vi "Sine_Trajectory.vi"(7 "Amplitude":dbl, 8 "Offset":dbl, 9 "Frequency (Hz)":dbl, 10 "Duration (s)":dbl, 11 "Period (s)":dbl) -> (3 "Profile":cluster{"time (s)":dbl, "setpoint":dbl}[](array[cluster]) {"setpoint" format="%.2f"; "time (s)" format="%.3f"})   [LabVIEW 2015]
uses:
  <vilib>/Analysis/NI_AALBase.lvlib
panel:
  out "XY Graph":cluster{dbl, dbl}[](graph)
  # "Here needs to be 0.001 or so"
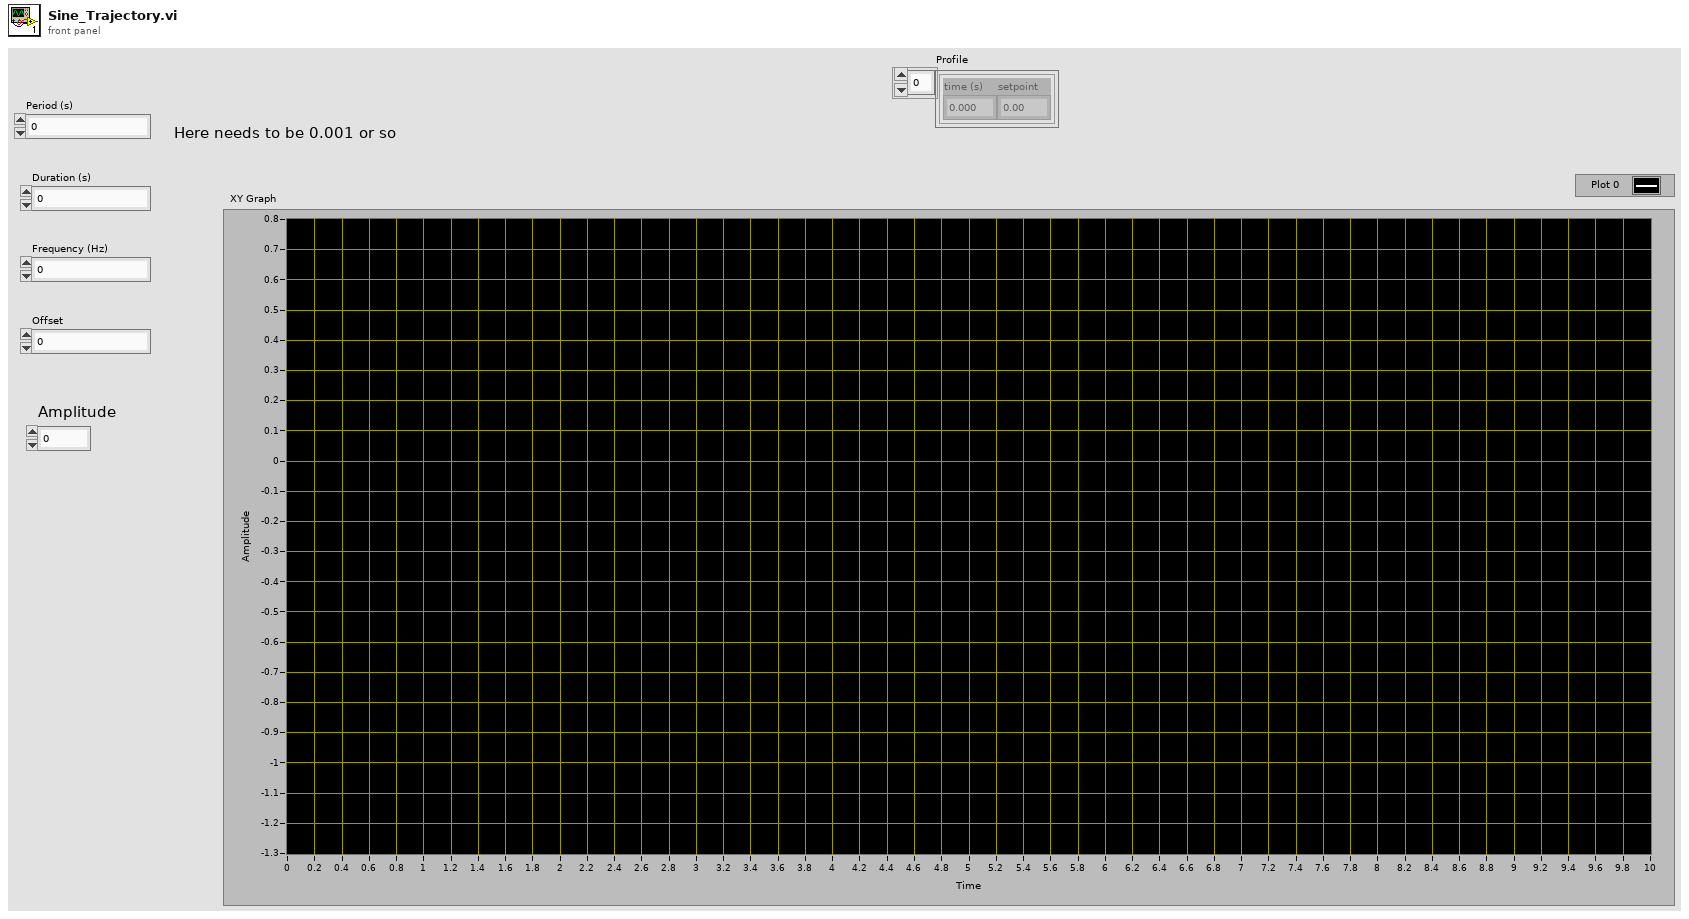
[diagram p1: front panel]
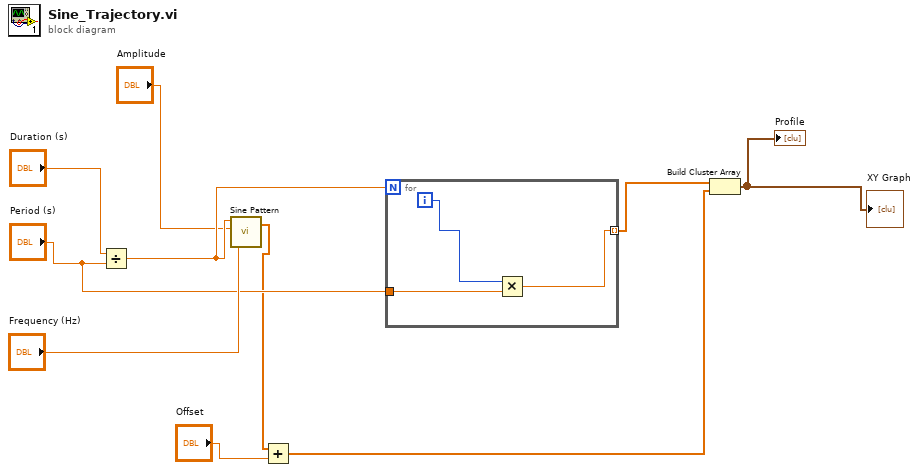
[diagram p0: block diagram]
diagram:
  n1 = Divide(x="Duration (s)", y="Period (s)") -> (x/y=w8:dbl)
  n2 = call <vilib>:"Sine Pattern.vi"("cycles"="Frequency (Hz)", "amplitude"="Amplitude", "samples"=w8) -> ("Sinusoidal Pattern"=w3:dbl[])  [unwired: 1 in, 1 out]
  n3 = Add(x=w3, y="Offset") -> (x+y=w2:dbl[])
  n4 = for {
    N: w8 -> [_]
    tunnel: [w11] -> w7 mode=indexing
    tunnel: "Period (s)" -> [w13]
    i -> [w12]
    n5 = Multiply(x=w12, y=w13) -> (x*y=w11:dbl)
  }
  n6 = Build Cluster Array(w7, w2) -> (→"XY Graph" →"Profile":cluster{dbl, dbl}[])
